vi "MagPS_eval_param_max.vi"(7 "admin_mode":bool, 9 "Current":dbl, 10 "x":dbl, 11 "Target Species":dbl) -> (0 "target_field_max":dbl, 1 "target_current_max":dbl, 2 "ramp_rate_max":dbl, 3 "target_frequency_max":dbl)   [LabVIEW 2019]
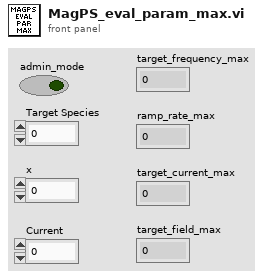
[diagram p1: front panel]
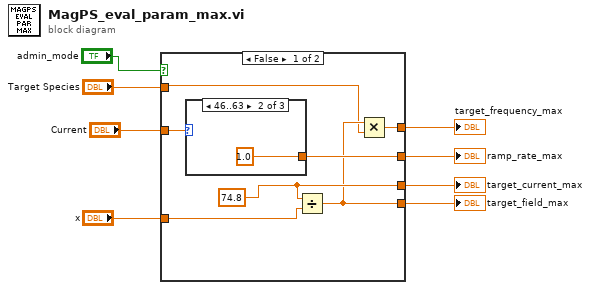
[diagram p0: block diagram]
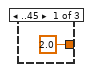
[diagram p2: hidden frame]
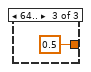
[diagram p3: hidden frame]
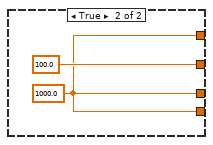
[diagram p4: hidden frame]
diagram:
  n1 = case shown="False" "admin_mode" {
    tunnel: [w12 w19] -> w1
    tunnel: [w15 100.0 ("Data Entry Limits:Maximum")] -> w6
    tunnel: "Current" -> [w14 _]
    tunnel: "x" -> [w13 _]
    tunnel: [w11 w19] -> w3
    tunnel: "Target Species" -> [w10 _]
    tunnel: [w9 w19] -> w4
    frame False {
      w12 = 74.8 ("Data Entry Limits:Maximum")
      n2 = case shown="46..63" w14 {
        tunnel: [2.0 ("Data Entry Limits:Maximum") 1.0 ("Data Entry Limits:Maximum") 0.5 ("Data Entry Limits:Maximum")] -> w15
        frame ..45 {
        }
        frame 46..63 {
        }
        frame 64.. {
        }
      }
      n3 = Divide(x=w12, y=w13) -> (x/y=w11:dbl)
      n4 = Multiply(x=w11, y=w10) -> (x*y=w9:dbl)
    }
    frame True {
      w19 = 1000.0 ("Data Entry Limits:Maximum")
    }
  }
  "ramp_rate_max" <- w6
  "target_frequency_max" <- w4
  "target_field_max" <- w3
  "target_current_max" <- w1
